vi "Exercise 5 Solution.vi"() -> ()   [LabVIEW 2019]
panel:
  out "Customer Data out":T1={"Element to Update"=enum."Age", "Name"="Adam", "Age"=23, "Is Married?"=TRUE, "Number of Updates"=8}
  in  "Is Married?":bool
  in  "Age":u8=23
  in  "Name":string="Adam"
  in  "Customer Data in":T1={"Element to Update"=enum."Age", "Name"="Adam", "Age"=0, "Is Married?"=TRUE, "Number of Updates"=7}
  # "Data to Update"
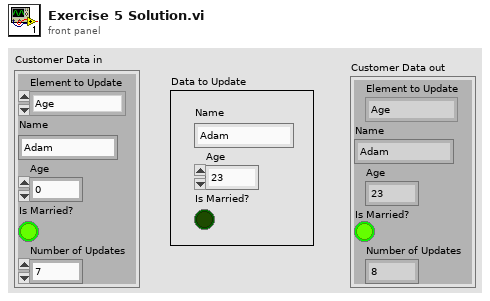
[diagram p1: front panel]
types:
  T1 = cluster{"Element to Update":enum16{"<None>", "Name", "Age", "Is Married?"}, "Name":string, "Age":u8, "Is Married?":bool, "Number of Updates":i32}
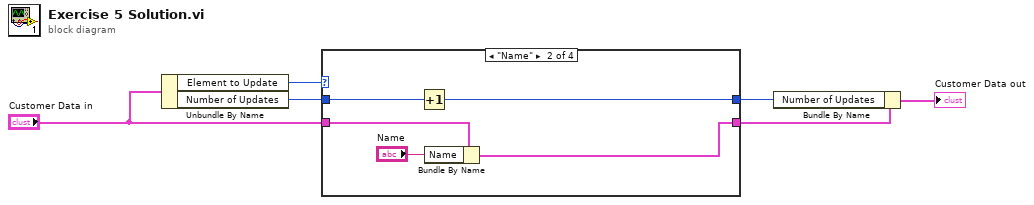
[diagram p0: block diagram]
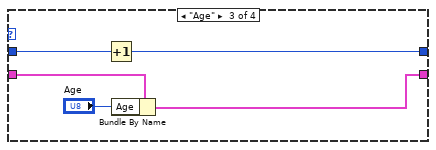
[diagram p3: hidden frame]
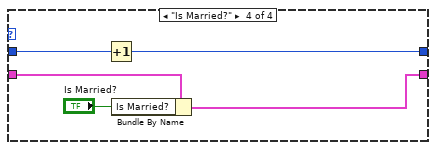
[diagram p4: hidden frame]
diagram:
  n1 = Unbundle By Name("Customer Data in") -> ("Element to Update"=w6:enum16{"<None>", "Name", "Age", "Is Married?"}, "Number of Updates"=w2:i32)
  n2 = case shown="\"Name\"" w6 {
    tunnel: "Customer Data in" -> [w8 w13 w18 w23]
    tunnel: [w8 w11 w17 w22] -> w4
    tunnel: w2 -> [w7 w10 w15 w20]
    tunnel: [w7 w9 w14 w19] -> w1
    frame "<None>", Default {
    }
    frame "Name" {
      n3 = Increment(x=w10) -> (x+1=w9:i32)
      n4 = Bundle By Name(cluster=w13, "Name"="Name") -> (w11:T1)
    }
    frame "Age" {
      n5 = Increment(x=w15) -> (x+1=w14:i32)
      n6 = Bundle By Name(cluster=w18, "Age"="Age") -> (w17:T1)
    }
    frame "Is Married?" {
      n7 = Increment(x=w20) -> (x+1=w19:i32)
      n8 = Bundle By Name(cluster=w23, "Is Married?"="Is Married?") -> (w22:T1)
    }
  }
  n9 = Bundle By Name(cluster=w4, "Number of Updates"=w1) -> (→"Customer Data out":T1)
